vi "Generate code.vi"(1 "Terms":T1, 3 "Diagram":refnum<vi>, 5 "XRef":refnum<vi>, 6 "State In":T5) -> (0 "Generated Code?":bool, 2 "State Out":T5, 4 "Reply":string[](array[string]))   [LabVIEW 2012, in "Array Dimension Array.xnode"]
uses:
  Array Dimension Array.xnode
  State.ctl
  <vilib>/XNodeSupport/XNodeTermIDPairs.ctl
  <vilib>/XNodeSupport/XNodeTermIDPair.ctl
  <vilib>/XNodeSupport/XNodeTermRef.ctl
  <vilib>/XNodeSupport/XNodeString.ctl
  <vilib>/Utility/miscctls.llb/LVPositionTypeDef.ctl
  VI Scripting/Scripting Tools/Scripting Tools.lvlib
  <vilib>/XNodeSupport/NI_XNodeSupport.lvlib
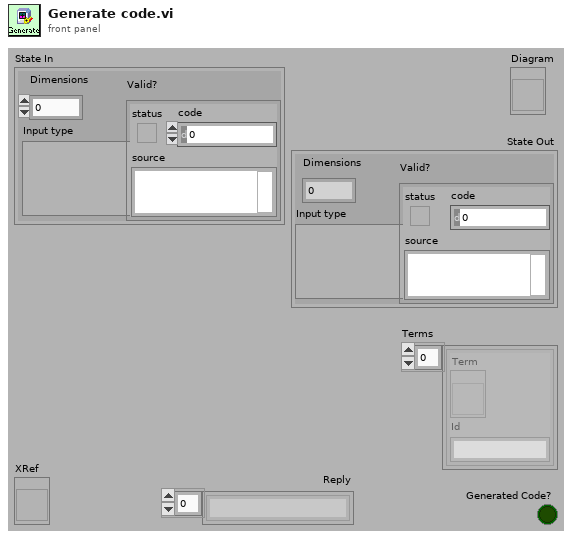
[diagram p1: front panel]
types:
  T1 = typedef "NI_XNodeSupport.lvlib/XNodeTermIDPairs.ctl" = T2[]
  T2 = typedef "NI_XNodeSupport.lvlib/XNodeTermIDPair.ctl" = cluster{"Term":T3, "Id":T4}
  T3 = typedef "NI_XNodeSupport.lvlib/XNodeTermRef.ctl" = refnum<vi>
  T4 = typedef "NI_XNodeSupport.lvlib/XNodeString.ctl" = string
  T5 = typedef "Array Dimension Array.xnode/State.ctl" = cluster{"Input type":variant, "Valid?":errorcluster, "Dimensions":i32}
  T6 = typedef "LVPositionTypeDef.ctl" = cluster{"Left":i32, "Top":i32}
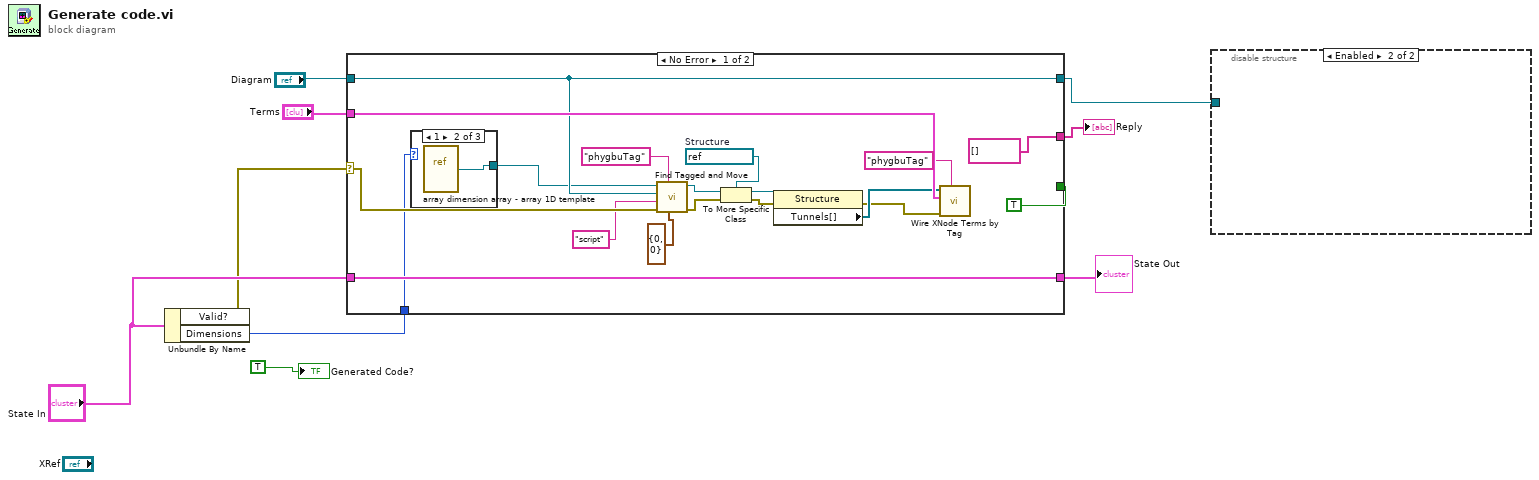
[diagram p0: block diagram]
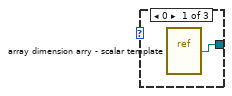
[diagram p2: hidden frame]
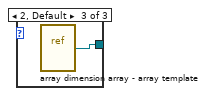
[diagram p3: hidden frame]
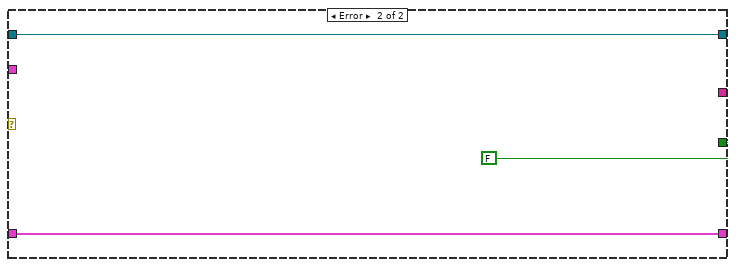
[diagram p4: hidden frame]
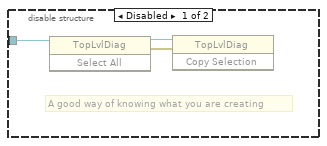
[diagram p5: hidden frame]
diagram:
  n1 = Unbundle By Name("State In") -> ("Valid?"=w2:errorcluster, "Dimensions"=w1:i32)
  n2 = case shown="No Error" w2 {
    selector: w2 -> [w21 _]
    tunnel: "State In" -> [w26 w34]
    tunnel: "Diagram" -> [w20 w32]
    tunnel: "Terms" -> [w25 _]
    tunnel: [w20 w32] -> w3
    tunnel: [string[] [] ("Reply") _] -> w4
    tunnel: [TRUE FALSE] -> _
    tunnel: [w26 w34] -> w6
    tunnel: w1 -> [w11 _]
    frame No Error {
      w23 = refnum<vi> refnum  # Structure
      n3 = case shown="1" w11 {
        tunnel: [w29 w30 w31] -> w10
        frame 0 {
          n4 = vi-ref "array dimension arry - scalar template.vi"() -> (w29:refnum<vi>)
        }
        frame 1 {
          n5 = vi-ref "array dimension array - array 1D template.vi"() -> (w30:refnum<vi>)
        }
        frame 2, Default {
          n6 = vi-ref "array dimension array - array template.vi"() -> (w31:refnum<vi>)
        }
      }
      n7 = call "Find Tagged and Move.vi"("position"=T6 {"Left"=0, "Top"=0}, "TagName"="phygbuTag", "error in"=w21, "TagValue"="script", "Destination Diagram"=w20, "VI Refnum"=w10) -> ("error out"=w15:errorcluster, "Moved Tagged object"=w16:refnum<vi>)  [unwired: 4 out]
      n8 = To More Specific Class(target class=w23, reference=w16, error in=w15) -> (specific class reference=w24:refnum<vi>, error out=w14:errorcluster)
      n9 = property class="Structure"(reference=w24, error in=w14) -> (error out=w13:errorcluster, "Tunnels[]"=w22:refnum<vi>[])  [unwired: 1 out]
      n10 = call "Wire XNode Terms by Tag.vi"("TagName"="phygbuTag", "error in (no error)"=w13, "Term Refs"=w25, "Source References"=w22) -> ()  [unwired: 8 out]
    }
    frame Error {
    }
  }
  "State Out" <- w6
  "Reply" <- w4
  n11 = disable-structure shown="Enabled" {
    disable-tunnel: w3 -> [w36 _]
    frame Disabled {
      # "A good way of knowing what you are creating"
      n12 = invoke class="TopLvlDiag" method="Select All"(reference=w36) -> (reference out=w37:refnum<vi>, error out=w35:errorcluster)  [unwired: 2 in, 1 out]
      n13 = invoke class="TopLvlDiag" method="Copy Selection"(reference=w37, error in=w35) -> ()  [unwired: 1 in, 3 out]
    }
    frame Enabled {
    }
  }
  "Generated Code?" <- TRUE
